vi "UTIL Piezo Feat_Filtered.vi"(4 "Init/Cont?":bool=TRUE, 6 "Filter Coefficients from File":dbl[][](array[numeric]), 7 "Piezo In":waveform(dbl)) -> (1 "Piezo Power":dbl format="%0.2f", 3 "Filtered Piezo Out":waveform(dbl))   [LabVIEW 2017]
doc: "This VI computed the r.m.s. power in the Piezo signal to serve as a surrogate fo EMG power in the task of sleep wake differentiation.\n\nInputs\n Piezo In Waveform\nOutputs\n Piezo Power DBL"
uses:
  <vilib>/Analysis/baseanly.llb/Mean (DBL).vi
  <vilib>/Analysis/3filter.llb/IIR Filter (DBL).vi
  <vilib>/Analysis/NI_AALBase.lvlib
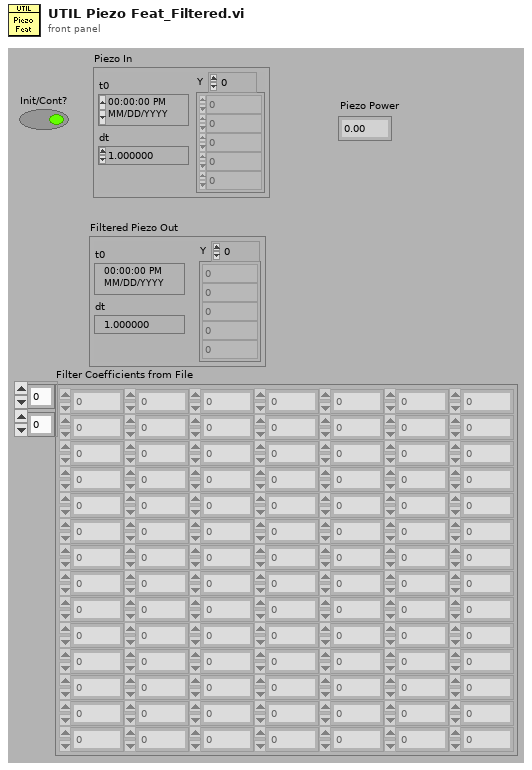
[diagram p1: front panel]
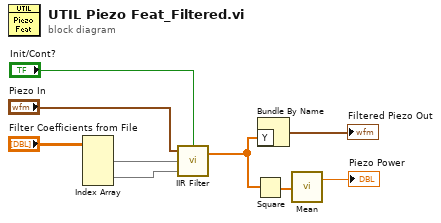
[diagram p0: block diagram]
diagram:
  n1 = Index Array(array="Filter Coefficients from File") -> (element #1=w5:dbl[], element #2=w4:dbl[])  [unwired: 4 in]
  n2 = call-poly <vilib>:"IIR Filter.vi"("init/cont (init:F)"="Init/Cont?", "Forward Coefficients"=w4, "Reverse Coefficients"=w5, "X"="Piezo In") -> ("Filtered X"=w1:dbl[])  [unwired: 1 out]
  n3 = Square(x=w1) -> (x^2=w9:dbl[])
  n4 = Bundle By Name("Y"=w1) -> (→"Filtered Piezo Out":waveform(dbl))  [unwired: 1 in]
  n5 = call-poly <vilib>:"Mean.vi"("X"=w9) -> ("mean"=→"Piezo Power":dbl)  [unwired: 1 out]
